vi "ScaleFactors.vi"(1 "data":i16, 2 "srcId":u8) -> (0 "dataOut":dbl)   [LabVIEW 2010]
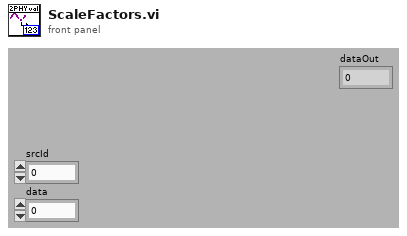
[diagram p1: front panel]
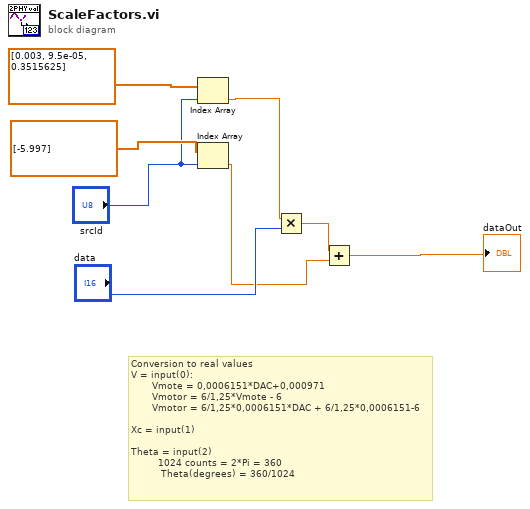
[diagram p0: block diagram]
diagram:
  # "Conversion to real values\nV = input(0): \n       Vmote = 0,0006151*DAC+0,000971\n       Vmotor = 6/1,25*Vmote - 6\n       Vmotor = 6/1,25*0,0006151*DAC + 6/1,25*0,0006151-6\n\nXc = input(1)\n\nTheta = input(2)\n         1024 counts = 2*Pi = 360\n          Theta(degrees) = 360/1024"
  n1 = Index Array(array=dbl[] [0.003, 9.5e-05, 0.3515625], index="srcId") -> (element=w8:dbl)
  n2 = Index Array(array=dbl[] [-5.997], index="srcId") -> (element=w3:dbl)
  n3 = Multiply(x=w8, y="data") -> (x*y=w6:dbl)
  n4 = Add(x=w6, y=w3) -> (x+y=→"dataOut":dbl)
